vi "Post-Install Custom Action.vi"(10 "Variant":variant) -> (0 "error out":errorcluster)   [LabVIEW 2019]
uses:
  <userlib>/_OpenG.lib/string/string.llb/Trim Whitespace (String)__ogtk.vi
  <vilib>/zip/NI_Unzip.lvlib
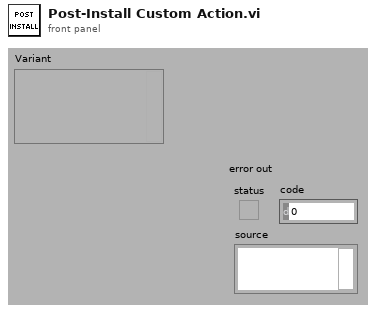
[diagram p1: front panel]
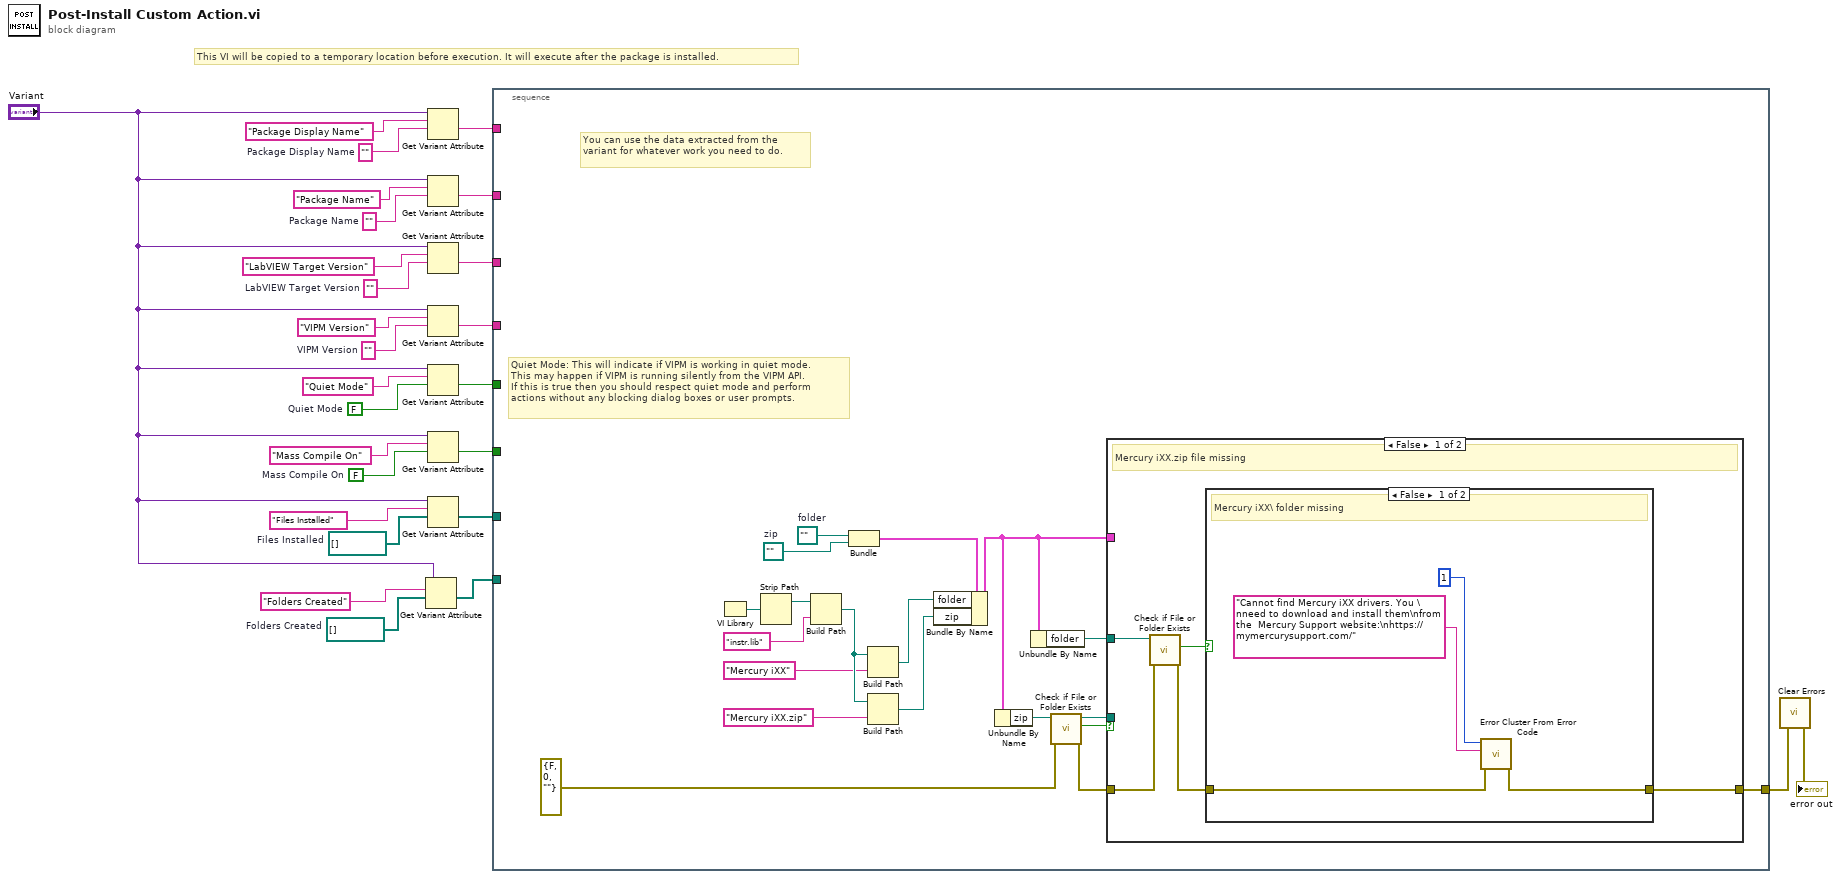
[diagram p0: block diagram]
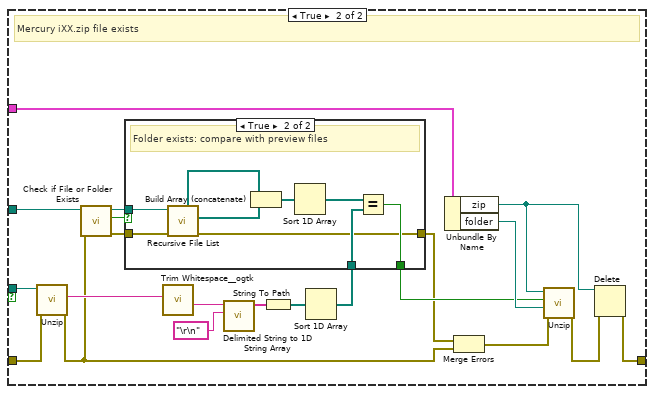
[diagram p3: hidden frame]
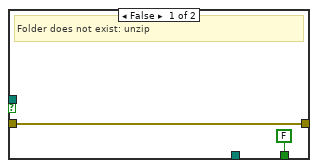
[diagram p4: hidden frame]
diagram:
  w3 = path[] []  # Folders Created
  w4 = path[] []  # Files Installed
  w10 = FALSE  # Mass Compile On
  w11 = ""  # Package Display Name
  w18 = FALSE  # Quiet Mode
  w21 = ""  # VIPM Version
  w23 = ""  # LabVIEW Target Version
  w25 = ""  # Package Name
  # "This VI will be copied to a temporary location before execution. It will execute after the package is installed."
  n1 = Get Variant Attribute(Variant="Variant", name="Folders Created", default value (empty Variant)=w3) -> (value=w8:path[])  [unwired: 1 in, 3 out]
  n2 = Get Variant Attribute(Variant="Variant", name="Package Display Name", default value (empty Variant)=w11) -> (value=w17:string)  [unwired: 1 in, 3 out]
  n3 = Get Variant Attribute(Variant="Variant", name="Package Name", default value (empty Variant)=w25) -> (value=w16:string)  [unwired: 1 in, 3 out]
  n4 = Get Variant Attribute(Variant="Variant", name="LabVIEW Target Version", default value (empty Variant)=w23) -> (value=w15:string)  [unwired: 1 in, 3 out]
  n5 = Get Variant Attribute(Variant="Variant", name="VIPM Version", default value (empty Variant)=w21) -> (value=w14:string)  [unwired: 1 in, 3 out]
  n6 = Get Variant Attribute(Variant="Variant", name="Quiet Mode", default value (empty Variant)=w18) -> (value=w13:bool)  [unwired: 1 in, 3 out]
  n7 = Get Variant Attribute(Variant="Variant", name="Mass Compile On", default value (empty Variant)=w10) -> (value=w12:bool)  [unwired: 1 in, 3 out]
  n8 = Get Variant Attribute(Variant="Variant", name="Files Installed", default value (empty Variant)=w4) -> (value=w7:path[])  [unwired: 1 in, 3 out]
  n9 = stacked-sequence {
    tunnel: w17 -> [_]
    tunnel: w16 -> [_]
    tunnel: w15 -> [_]
    tunnel: w14 -> [_]
    tunnel: w13 -> [_]
    tunnel: w12 -> [_]
    tunnel: w7 -> [_]
    tunnel: w8 -> [_]
    tunnel: [w46] -> w2
    frame #0 {
      w35 = path ""  # zip
      w34 = path ""  # folder
      # "Quiet Mode: This will indicate if VIPM is working in quiet mode.\nThis may happen if VIPM is running silently from the VIPM API.\nIf this is true then you should respect quiet mode and perform\nactions without any blocking dialog boxes or user prompts."
      # "You can use the data extracted from the variant for whatever work you need to do."
      n10 = VI Library() -> (path=w29:path)
      n11 = Strip Path(path=w29) -> (stripped path=w30:path)  [unwired: 1 out]
      n12 = Build Path(base path=w30, name or relative path="instr.lib") -> (appended path=w33:path)
      n13 = Bundle("folder"=w34, "zip"=w35) -> (w36:cluster{"folder":path, "zip":path})  [unwired: 1 in]
      n14 = Build Path(base path=w33, name or relative path="Mercury iXX") -> (appended path=w37:path)
      n15 = Build Path(base path=w33, name or relative path="Mercury iXX.zip") -> (appended path=w38:path)
      n16 = Bundle By Name(cluster=w36, "folder"=w37, "zip"=w38) -> (w41:cluster{"folder":path, "zip":path})
      n17 = Unbundle By Name(w41) -> ("zip"=w39:path)
      n18 = Unbundle By Name(w41) -> ("folder"=w40:path)
      n19 = call <vilib>:"Check if File or Folder Exists.vi"("error in (no error)"=errorcluster {"status"=FALSE, "code"=0, "source"=""}, "path"=w39) -> ("error out"=w43:errorcluster, "file or folder exists?"=w44:bool, "dup path"=w42:path)  [unwired: 7 in]
      n20 = case shown="False" w44 {
        tunnel: [w47 w77] -> w46
        tunnel: w40 -> [w51 w76]
        tunnel: w41 -> [_ w75]
        tunnel: w42 -> [_ w68]
        tunnel: w43 -> [w50 w66]
        frame False {
          # "Mercury iXX.zip file missing"
          n21 = call <vilib>:"Check if File or Folder Exists.vi"("error in (no error)"=w50, "path"=w51) -> ("error out"=w48:errorcluster, "file or folder exists?"=w49:bool)  [unwired: 7 in, 1 out]
          n22 = case shown="False" w49 {
            tunnel: w48 -> [w55 w56]
            tunnel: [w52 w56] -> w47
            frame False {
              # "Mercury iXX\\ folder missing"
              n23 = call <vilib>:"Error Cluster From Error Code.vi"("error in (no error)"=w55, "error message (\"\")"="Cannot find Mercury iXX drivers. You \nneed to download and install them\nfrom the  Mercury Support website:\nhttps://mymercurysupport.com/" ("message"), "error code (0)"=1) -> ("error out"=w52:errorcluster)  [unwired: 6 in]
            }
            frame True {
              # "validate if contents are ok?"
              # "Mercury iXX\\ folder exists"
            }
          }
        }
        frame True {
          # "Mercury iXX.zip file exists"
          n24 = call <vilib>:"Unzip.vi"("error in (no error)"=w66, "Zip file"=w68) -> ("error out"=w57:errorcluster, "Preview"=w70:string)  [unwired: 7 in, 1 out]
          n25 = call <vilib>:"Check if File or Folder Exists.vi"("error in (no error)"=w57, "path"=w76) -> ("error out"=w60:errorcluster, "file or folder exists?"=w63:bool, "dup path"=w67:path)  [unwired: 7 in]
          n26 = call-poly <userlib>:"Trim Whitespace__ogtk.vi"("String in"=w70) -> ("String out"=w69:string)  [unwired: 6 in]
          n27 = call <vilib>:"Delimited String to 1D String Array.vi"("delimiter"="\r\n", "delimited string"=w69) -> ("string array"=w72:string[])  [unwired: 9 in]
          n28 = String To Path(string=w72) -> (path=w71:path[])
          n29 = Sort 1D Array(array=w71) -> (sorted array=w65:path[])
          n30 = case shown="True" w63 {
            tunnel: w67 -> [_ w85]
            tunnel: w65 -> [_ w84]
            tunnel: [FALSE w83] -> w64
            tunnel: w60 -> [w78 w81]
            tunnel: [w78 w80] -> w59
            frame False {
              # "Folder does not exist: unzip"
            }
            frame True {
              # "Folder exists: compare with preview files"
              n31 = call <vilib>:"Recursive File List.vi"("error in (no error)"=w81, "Folder Path"=w85) -> ("error out"=w80:errorcluster, "All Files in Dir"=w87:path[], "All Folders"=w88:path[])  [unwired: 5 in, 2 out]
              n32 = Build Array (concatenate)(w88, w87) -> (w86:path[])
              n33 = Sort 1D Array(array=w86) -> (sorted array=w82:path[])
              n34 = Equal?(x=w82, y=w84) -> (x = y?=w83:bool)
            }
          }
          n35 = Unbundle By Name(w75) -> ("zip"=w61:path, "folder"=w74:path)
          n36 = Merge Errors(w59, w57) -> (w58:errorcluster)
          n37 = call <vilib>:"Unzip.vi"("error in (no error)"=w58, "Target directory (same as Zip file if empty)"=w74, "Preview only?"=w64, "Zip file"=w61) -> ("error out"=w62:errorcluster)  [unwired: 5 in, 2 out]
          n38 = Delete(path (use dialog)=w61, error in=w62) -> (error out=w77:errorcluster)  [unwired: 3 in, 2 out]
        }
      }
    }
  }
  n39 = call <vilib>:"Clear Errors.vi"("error in (no error)"=w2) -> ("error out"=→"error out":errorcluster)  [unwired: 5 in, 1 out]
